vi "getDeviceByName.vi"(8 "error in (no error)":errorcluster, 10 "deviceName":string, 11 "DeviceArray in":refnum<class "DeviceArray.lvclass">) -> (0 "error out":errorcluster, 1 "found?":bool, 2 "device.lvclass":refnum<class "device.lvclass">, 3 "DeviceArray out":refnum<class "DeviceArray.lvclass">)   [LabVIEW 2011, in "Tools.lvlib" / "DatabaseHelpers.lvlib" / "DeviceArray.lvclass"]
uses:
  DeviceArray.lvclass
  device/device.lvclass
  DeviceArray.lvclass/DeviceArray.ctl
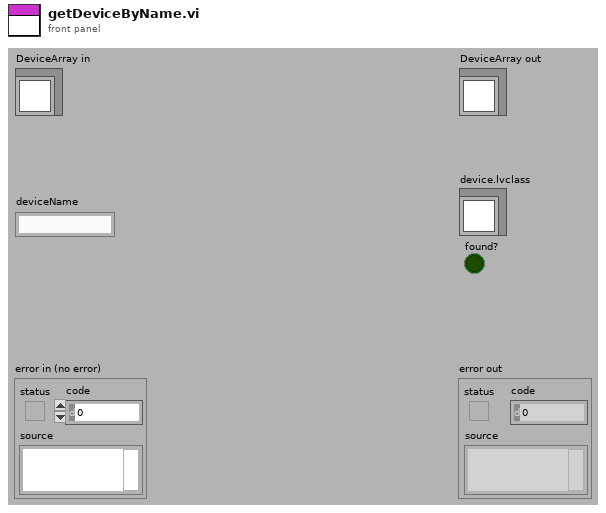
[diagram p1: front panel]
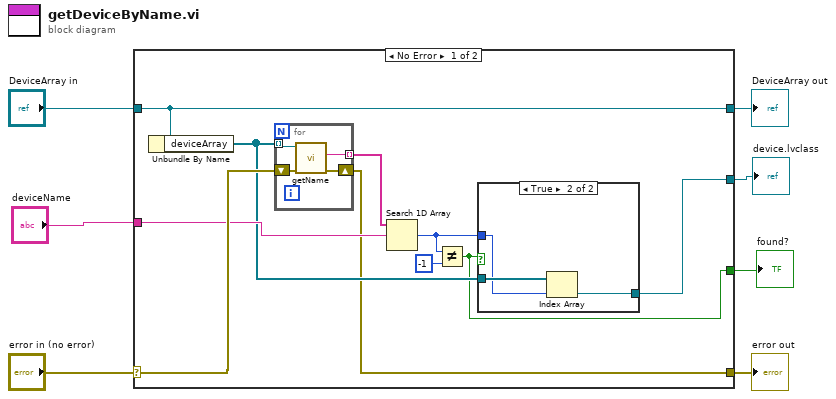
[diagram p0: block diagram]
diagram:
  n1 = case shown="No Error" "error in (no error)" {
    selector: "error in (no error)" -> [w16 w26]
    tunnel: [w9 w26] -> w6
    tunnel: [w17 w25] -> w4
    tunnel: "DeviceArray in" -> [w17 w25]
    tunnel: "deviceName" -> [w14 _]
    tunnel: [w11 _] -> w2
    tunnel: [w10 _] -> w1
    frame No Error {
      n2 = Unbundle By Name(w17) -> ("deviceArray"=w12:refnum<class "device.lvclass">[])
      n3 = for {
        tunnel: w12 -> [w24] mode=indexing
        tunnel: [w22] -> w15 mode=indexing
        shift-right: [w21] -> w9
        shift-left: w16 -> [w23]
        n4 = call "getName.vi"("error in (no error)"=w23, "device.lvclass in"=w24) -> ("error out"=w21:errorcluster, "name"=w22:string)  [unwired: 7 in, 1 out]
      }
      n5 = Search 1D Array(1D array=w15, element=w14) -> (index of element=w8:i32)  [unwired: 1 in]
      n6 = Not Equal?(x=w8, y=-1) -> (x != y?=w10:bool)
      n7 = case shown="True" w10 {
        tunnel: w12 -> [_ w20]
        tunnel: [_ w19] -> w11
        tunnel: w8 -> [_ w18]
        frame False {
        }
        frame True {
          n8 = Index Array(array=w20, index=w18) -> (element=w19:refnum<class "device.lvclass">)
        }
      }
    }
    frame Error {
    }
  }
  "error out" <- w6
  "DeviceArray out" <- w4
  "device.lvclass" <- w2
  "found?" <- w1
